vi "PCO_Live.vi"(7 "Message Data":variant, 8 "entrée d'erreur (pas d'erreur)":errorcluster, 9 "Display loop":refnum<queue>, 10 "dup Message Queue":refnum<queue>, 11 "Camera en entrée":refnum<class "Camera.lvclass">) -> (0 "sortie d'erreur":errorcluster, 3 "Camera en sortie":refnum<class "Camera.lvclass">)   [LabVIEW 2026]
uses:
  QMH/Message Queue/Message Cluster.ctl
  <instrlib>/PCO_SDK/File Group 0/vi.lib/Excelitas PCO GmbH/pco.labview/camera/Camera.lvclass
  Controls/PCO_Config.ctl
  Controls/TypeDef_FGV.ctl
  QMH/Message Queue/Enqueue Message (Single).vi
  QMH/Message Queue/Message Queue.lvlib
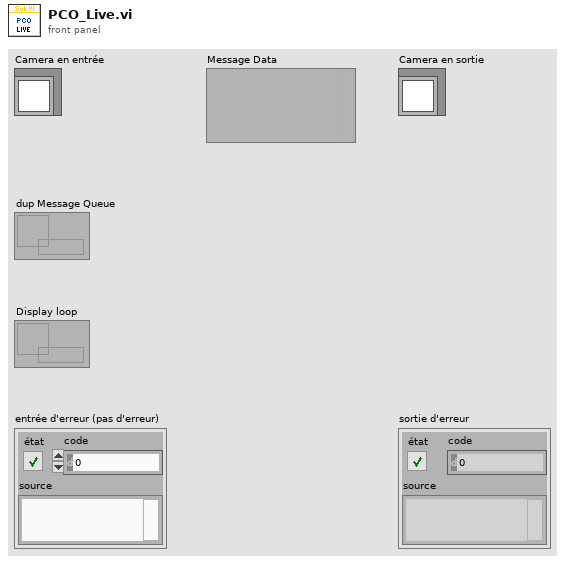
[diagram p1: front panel]
types:
  T1 = typedef "PCO_Config.ctl" = cluster{"Exposure time (s)":dbl, "TriggerMode":u16, "ROI X0":u16, "ROI Y0":u16, "ROI X1":u16, "ROI Y1":u16, "Binning":u8}
  T2 = enum16{"sequence", "sequence non blocking", "ring buffer", "fifo", "sequence_dpcore", "sequence_non_blocking_dpcore", "ring_buffer_dpcore", "fifo_dpcore", "tif", "multitif", "pcoraw", "b16", "dicom", "multidicom", "camram_ring", "camram_segment"}
  T3 = typedef "TypeDef_FGV.ctl" = enum16{"Initialize", "Write", "Read"}
  T4 = enum16{"Undefined", "Mono8", "Mono16", "BGRA8", "RGBA8", "BGRA16", "RGBA16", "CompressedMono8"}
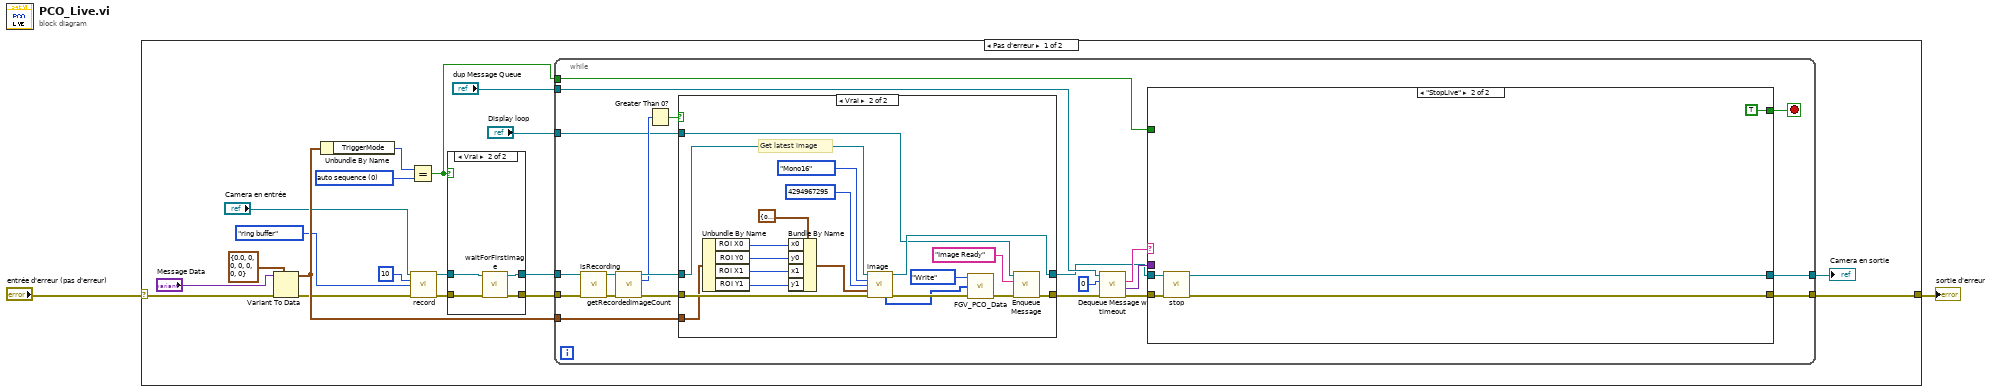
[diagram p0: block diagram]
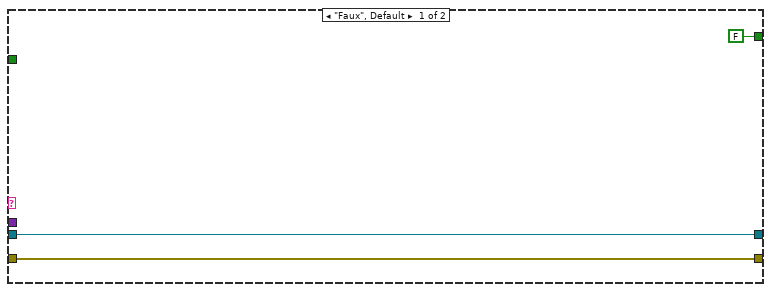
[diagram p2: hidden frame]
diagram:
  n1 = case shown="Pas d'erreur" "entrée d'erreur (pas d'erreur)" {
    selector: "entrée d'erreur (pas d'erreur)" -> [w4 w78]
    tunnel: [w17 w78] -> w2
    frame No Error {
      w10 = u16 0 items=["auto sequence", "software trigger", "external exposure start", "external exposure control"] ("TriggerMode")
      n2 = Variant To Data(error in=w4, type=T1 {"Exposure time (s)"=0.0, "TriggerMode"=0, "ROI X0"=0, "ROI Y0"=0, "ROI X1"=0, "ROI Y1"=0, "Binning"=0} ("PCO_Config"), Variant="Message Data") -> (data=w15:T1, error out=w9:errorcluster)
      n3 = Unbundle By Name(w15) -> ("TriggerMode"=w11:u16)
      n4 = Equal?(x=w11, y=w10) -> (x = y?=w3:bool)
      n5 = call-dynamic "record.vi"("Camera in"="Camera en entrée", "num_images"=u32 10 ("dwImgCount"), "record_mode"=T2."ring buffer", "error in (no error)"=w9) -> ("Camera out"=w20:refnum<class "Camera.lvclass">, "error out"=w19:errorcluster)  [unwired: 10 in]
      n6 = case shown="Vrai" w3 {
        tunnel: w19 -> [w72 w77]
        tunnel: w20 -> [w73 w76]
        tunnel: [w73 w75] -> w14
        tunnel: [w72 w74] -> w13
        frame False {
        }
        frame True {
          n7 = call-dynamic "waitForFirstImage.vi"("error in (no error)"=w77, "Camera in"=w76) -> ("error out"=w74:errorcluster, "Camera out"=w75:refnum<class "Camera.lvclass">)  [unwired: 8 in]
        }
      }
      n8 = while {
        tunnel: w13 -> [w36]
        tunnel: w14 -> [w35]
        tunnel: w15 -> [w34]
        tunnel: "dup Message Queue" -> [w32]
        tunnel: "Display loop" -> [w30]
        tunnel: [w26] -> w17
        tunnel: [w25] -> w18
        tunnel: w3 -> [w22]
        stop <- w24 stop-if-true
        n9 = call-dynamic "isRecording.vi"("Camera in"=w35, "error in (no error)"=w36) -> ("Camera out"=w42:refnum<class "Camera.lvclass">, "error out"=w41:errorcluster)  [unwired: 11 in, 1 out]
        n10 = call-dynamic "getRecordedImageCount.vi"("Camera in"=w42, "error in (no error)"=w41) -> ("Camera out"=w39:refnum<class "Camera.lvclass">, "recorded_image_count"=w37:u32, "error out"=w40:errorcluster)  [unwired: 11 in]
        n11 = Greater Than 0?(x=w37) -> (x > 0?=w38:bool)
        n12 = case shown="Vrai" w38 {
          tunnel: [w51 w57] -> w33
          tunnel: w40 -> [w51 w68]
          tunnel: w39 -> [w52 w67]
          tunnel: [w52 w66] -> w27
          tunnel: w34 -> [_ w65]
          tunnel: w30 -> [_ w59]
          frame False {
          }
          frame True {
            # "Get latest image"
            n13 = Unbundle By Name(w65) -> ("ROI X0"=w64:u16, "ROI Y0"=w63:u16, "ROI X1"=w62:u16, "ROI Y1"=w61:u16)
            n14 = Bundle By Name(cluster=cluster{"x0":u64, "y0":u64, "x1":u64, "y1":u64} {"x0"=0, "y0"=0, "x1"=0, "y1"=0} ("roi"), "x0"=w64, "y0"=w63, "x1"=w62, "y1"=w61) -> (w69:cluster{"x0":u64, "y0":u64, "x1":u64, "y1":u64})
            n15 = call-dynamic "image.vi"("Camera in"=w67, "data_format"=T4."Mono16", "image_index"=u32 4294967295 ("dwImgIdx"), "roi"=w69, "error in (no error)"=w68) -> ("Camera out"=w66:refnum<class "Camera.lvclass">, "raw_image (U16)"=w53:u16[][], "error out"=w55:errorcluster)  [unwired: 2 in, 6 out]
            n16 = call "FGV_PCO_Data.vi"("error in"=w55, "Data"=w53, "Action"=TypeDef_FGV."Write") -> ("error out"=w54:errorcluster)  [unwired: 1 in, 1 out]
            n17 = call-poly "Enqueue Message.vi"("error in (no error)"=w54, "Message"="Image Ready", "Message Queue"=w59) -> ("error out"=w57:errorcluster)  [unwired: 7 in, 1 out]
          }
        }
        n18 = call "Dequeue Message w timeout.vi"("entrée d'erreur (pas d'erreur)"=w33, "timeout en ms (-1)"=0, "Message Queue"=w32) -> ("sortie d'erreur"=w29:errorcluster, "Message Data"=w28:variant, "Message"=w31:string)  [unwired: 5 in, 1 out]
        n19 = case shown="\"StopLive\"" w31 {
          tunnel: w29 -> [w44 w49]
          tunnel: w28 -> [_ _]
          tunnel: w27 -> [w45 w50]
          tunnel: [w44 w48] -> w26
          tunnel: [w45 w47] -> w25
          tunnel: [FALSE TRUE] -> w24
          tunnel: w22 -> [_ _]
          frame "Faux", Default {
          }
          frame "StopLive" {
            n20 = call-dynamic "stop.vi"("error in (no error)"=w49, "Camera in"=w50) -> ("error out"=w48:errorcluster, "Camera out"=w47:refnum<class "Camera.lvclass">)  [unwired: 8 in]
          }
        }
      }
      "Camera en sortie" <- w18
    }
    frame Error {
    }
  }
  "sortie d'erreur" <- w2
